vi "Owl429_TxAcyclicTransferConfig_getName.vi"(8 "error in (no error)":errorcluster, 11 "acyclic config handle":u32) -> (0 "error out":errorcluster, 2 "label":string, 3 "acyclic config handle":u32)   [LabVIEW 2015, in "AIT 429 System Explorer.lvlib"]
doc: "Gets the name of the label field for the label transfer.\n\nReturns:\nThe name string."
uses:
  AIT 429 System Explorer.lvlib
  <userlib>/ARINC-429/Owl429.lvlib
  owl429.dll
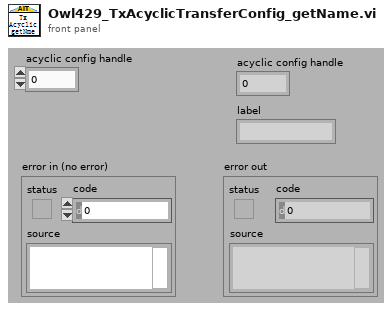
[diagram p1: front panel]
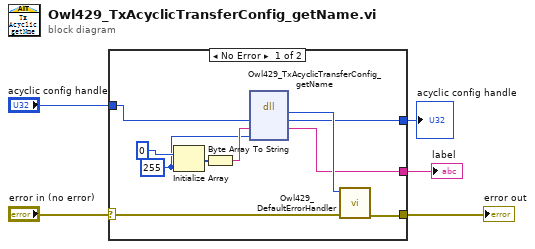
[diagram p0: block diagram]
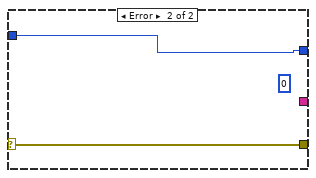
[diagram p2: hidden frame]
diagram:
  n1 = case shown="No Error" "error in (no error)" {
    selector: "error in (no error)" -> [w13 w17]
    tunnel: [w12 w17] -> w4
    tunnel: "acyclic config handle" -> [w14 w16]
    tunnel: [w11 w16] -> w2
    tunnel: [w10 _] -> w1
    frame No Error {
      w6 = 255 ("dimension size")
      n2 = Initialize Array(u8 0, w6) -> (w8:u8[])
      n3 = Byte Array To String(unsigned byte array=w8) -> (string=w7:string)
      n4 = dll-call lib="owl429.*" fn="Owl429_TxAcyclicTransferConfig_getName" ("429owl.*:Owl429_TxScheduledLabelConfig_getLabel")("label config handle"=w14, "label"=w7, "size"=w6) -> ("return type"=w15:i32, "label config handle"=w11:u32, "label"=w10:string)  [unwired: 4 in, 2 out]
      n5 = call <userlib>:"Owl429_DefaultErrorHandler.vi"("error in (no error)"=w13, "error code"=w15) -> ("error out"=w12:errorcluster)  [unwired: 9 in]
    }
    frame Error {
      (unwired) u8 0 ("label")
    }
  }
  "error out" <- w4
  "acyclic config handle" <- w2
  "label" <- w1
